vi "Add Breakpoints to all Nodes.vi"(8 "error in":errorcluster, 11 "VI Refnum In":refnum<vi>) -> (0 "error out":errorcluster, 3 "VI Refnum Out":refnum<vi>)   [LabVIEW 2020]
doc: "Add breakpoints to all nodes of the active VI."
uses:
  <vilib>/Utility/traverseref.llb/TRef TravTarget.ctl
  src/Type Definitions/Class Name--enum.ctl
  <vilib>/Utility/miscctls.llb/LVBreakpointStatusEnum.ctl
  <vilib>/Utility/traverseref.llb/VI Scripting - Traverse.lvlib
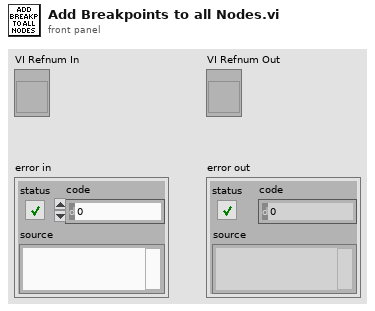
[diagram p1: front panel]
types:
  T1 = typedef "Class Name--enum.ctl" = enum16{"Node", "Wire"}
  T2 = typedef "TRef TravTarget.ctl" = enum16{"FP", "BD", "Other"}
  T3 = typedef "LVBreakpointStatusEnum.ctl" = enum8{"Cleared Break", "Enabled Break", "Disabled Break"}
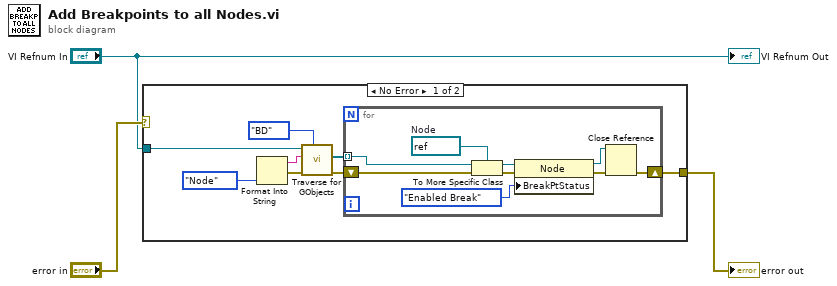
[diagram p0: block diagram]
diagram:
  n1 = case shown="No Error" "error in" {
    selector: "error in" -> [_ w21]
    tunnel: [w11 w21] -> w2
    tunnel: "VI Refnum In" -> [w4 _]
    frame No Error {
      n2 = Format Into String(Class_Name--enum."Node" ("input 1")) -> (resulting string=w8:string, error out=w10:errorcluster)  [unwired: 3 in]
      n3 = call <vilib>:"Traverse for GObjects.vi"("Traverse Target"=TRef_TravTarget."BD", "error in (no error)"=w10, "Class Name"=w8, "VI Refnum"=w4) -> ("error out"=w9:errorcluster, "References"=w5:refnum<vi>[])  [unwired: 4 in, 2 out]
      n4 = for {
        tunnel: w5 -> [w16] mode=indexing
        shift-right: [w17] -> w11
        shift-left: w9 -> [w20]
        w12 = refnum<vi> refnum  # Node
        n5 = To More Specific Class(target class=w12, reference=w16, error in=w20) -> (specific class reference=w15:refnum<vi>, error out=w19:errorcluster)
        n6 = property class="Node"(reference=w15, error in=w19, "BreakPtStatus"=LVBreakpointStatusEnum."Enabled Break" ("Breakpoint Status")) -> (reference out=w14:refnum<vi>, error out=w18:errorcluster)
        n7 = Close Reference(reference=w14, error in (no error)=w18) -> (error out=w17:errorcluster)
      }
    }
    frame Error {
      # "Pass error without further action"
    }
  }
  "error out" <- w2
  "VI Refnum Out" <- "VI Refnum In"
